vi "Set_ShutterTimingMode.vi"(8 "error in":errorcluster, 10 "ShutterTimingMode":T1=1 items=["Normal"=1, "AlwaysClosed"=2, "AlwaysOpen"=3, "OpenBeforeTrigger"=4], 11 "camera handle in":u64) -> (0 "error out":errorcluster, 3 "camera handle out":u64)   [LabVIEW 2014, in "PICam.lvlib"]
doc: "PicamShutterTimingMode_\nNormal\nThe shutter only opens during exposure time.\nNOTE: During PicamReadoutControlMode_Kinetics\nreadout, the shutter stays open while storing frames.\n\nPicamShutterTimingMode_\nAlwaysClosed\nThe shutter is always closed.\nNOTE: This mode is also valid when not acquiring data.\n\nPicamShutterTimingMode_\nAlwaysOpen\nThe shutter is always open.\nNOTE: This mode is also valid when not acquiring data.\n\nPicamShutterTimingMode_\nOpenBeforeTrigger\nThe shutter opens ahead of time while waiting for a trigger.\nThis is different from PicamShutterTimingMode_Normal\nwhere the shutter opens in reaction to a trigger."
uses:
  PICam.lvlib
  Ctrls/ShutterTimingMode.ctl
  Picam32.dll
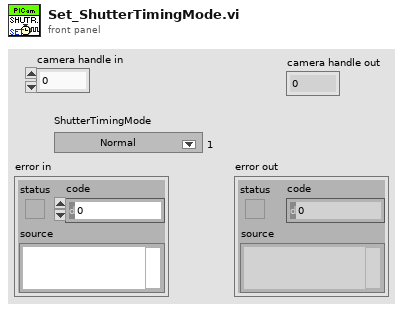
[diagram p1: front panel]
types:
  T1 = typedef "PICam.lvlib/ShutterTimingMode.ctl" = u32
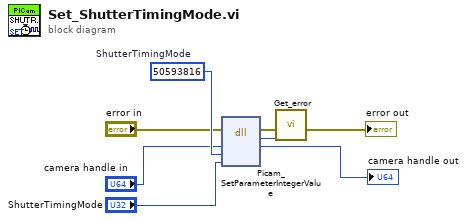
[diagram p0: block diagram]
diagram:
  w4 = u32 50593816  # ShutterTimingMode
  n1 = dll-call lib="Picam32.dll" fn="Picam_SetParameterIntegerValue"(error in="error in", "camera"="camera handle in", "PicamParameter"=w4, "ShutterTimingMode"="ShutterTimingMode") -> (error out=w8:errorcluster, "return type"=w7:i32, "camera"=→"camera handle out":u64)  [unwired: 4 in, 1 out]
  n2 = call "Get_error.vi"("PICam_Error"=w7, "error in (no error)"=w8) -> ("error out"=→"error out":errorcluster)  [unwired: 9 in]
